vi "Stop User Event_Algo.vi"(8 "error in (no error)":errorcluster, 11 "Algorithm in":refnum<class "Algorithm.lvclass">) -> (0 "error out":errorcluster, 3 "Algorithm out":refnum<class "Algorithm.lvclass">)   [LabVIEW 2015]
uses:
  <vilib>/event_ctls.llb/usereventprio.ctl
  FrameworkOverrides/Algorithm.lvclass
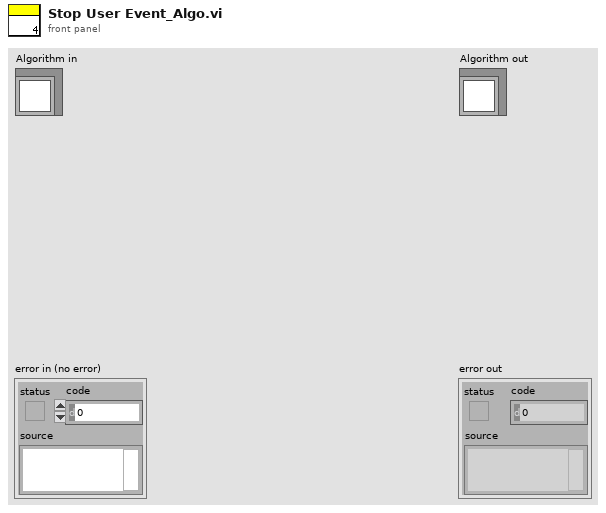
[diagram p1: front panel]
types:
  T1 = typedef "usereventprio.ctl" = enum32{"high priority", "normal priority"}
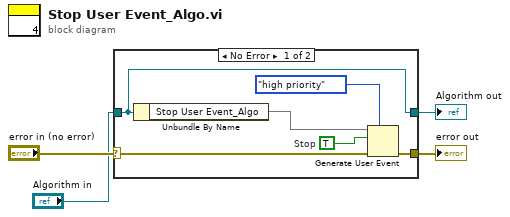
[diagram p0: block diagram]
diagram:
  n1 = case shown="No Error" "error in (no error)" {
    selector: "error in (no error)" -> [w7 w12]
    tunnel: [w6 w12] -> w3
    tunnel: [w10 w11] -> w1
    tunnel: "Algorithm in" -> [w10 w11]
    frame No Error {
      w8 = TRUE  # Stop
      n2 = Unbundle By Name(w10) -> ("Stop User Event_Algo"=w9)
      n3 = Generate User Event(priority (normal)=usereventprio."high priority", user event=w9, event data cluster=w8, error in=w7) -> (error out=w6:errorcluster)  [unwired: 1 out]
    }
    frame Error {
    }
  }
  "error out" <- w3
  "Algorithm out" <- w1
